vi "esp301 set home.vi"(7 "Seperator in":string, 8 "error in (no error)":errorcluster, 9 "Args":string[](array[string]), 10 "String":string, 11 "ESP301 in":refnum<class "ESP301.lvclass">) -> (0 "error out":errorcluster, 2 "new commands":string, 3 "ESP301 out":refnum<class "ESP301.lvclass">)   [LabVIEW 2020, in "ESP301.lvclass"]
uses:
  ESP301.lvclass
  ESP301.lvclass/ESP301.ctl
  shared/CompressAndUpdate(Poly)/CompressAndUpdate(Numeric).vi
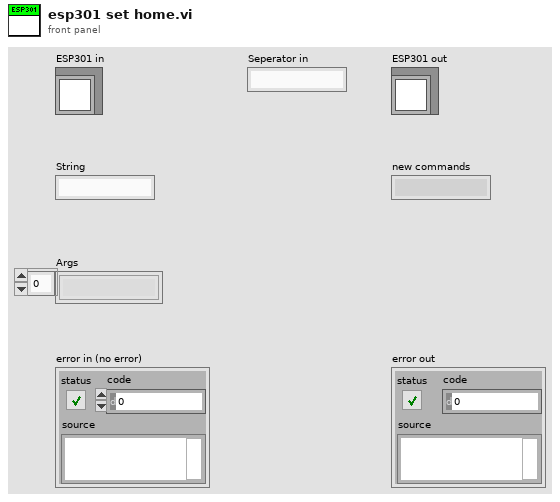
[diagram p1: front panel]
types:
  T1 = cluster{"Axis 1":cluster{"Value":dbl, "Min":dbl, "Max":dbl, "StepSize":dbl, "Tolerance":dbl, "ValueActual":dbl}, "Axis 2":cluster{"Value":dbl, "Min":dbl, "Max":dbl, "StepSize":dbl, "Tolerance":dbl, "ValueActual":dbl}, "Axis 3":cluster{"Value":dbl, "Min":dbl, "Max":dbl, "StepSize":dbl, "Tolerance":dbl, "ValueActual":dbl}}
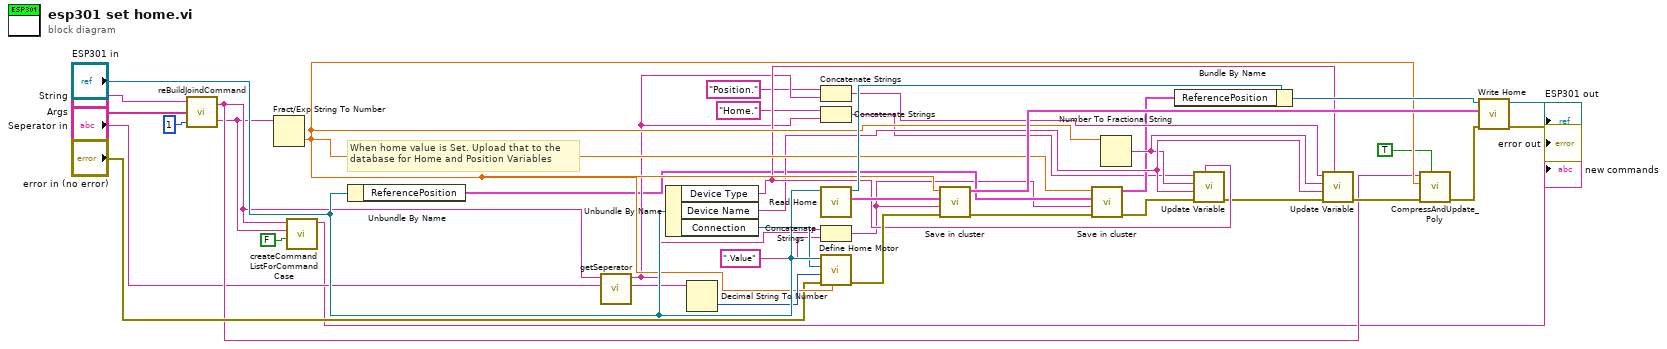
[diagram p0: block diagram]
diagram:
  # "When home value is Set. Upload that to the\ndatabase for Home and Position Variables"
  n1 = call "reBuildJoindCommand.vi"("number of group elements (0)"=1, "Args"="Args", "Command 2"="String") -> ("Arg"=w10:string, "Command"=w18:string)
  n2 = Fract/Exp String To Number(string=w10) -> (number=w28:dbl)  [unwired: 3 in, 1 out]
  n3 = call "createCommandListForCommandCase.vi"("immediate Check (only once)"=FALSE, "setvalue"=w10, "command"=w18) -> ("new commands"=→"new commands":string)  [unwired: 8 in]
  n4 = Unbundle By Name("ESP301 in") -> ("ReferencePosition"=w16:T1)
  n5 = call "getSeperator.vi"("Channel Seperator (\"\")"="Seperator in", "Command"=w18) -> ("Channel"=w8:string, "Seperator (e.g. \"Channel1\")"=w23:string)  [unwired: 8 in]
  n6 = Unbundle By Name("ESP301 in") -> ("Device Type"=w26:string, "Device Name"=w25:string, "Connection"=w29:refnum<visa-resource-name>)
  n7 = Decimal String To Number(string=w8) -> (number=w30:i32)  [unwired: 2 in, 1 out]
  n8 = Concatenate Strings("Position." ("string"), w23) -> (w22:string)
  n9 = Concatenate Strings("Home." ("string"), w23) -> (w12:string)
  n10 = call "Read Home.vi"("ESP301 in"="ESP301 in") -> ("Home"=w34:T1, "ESP301 out"=w32:refnum<class "ESP301.lvclass">)  [unwired: 8 in, 1 out]
  n11 = Concatenate Strings(w23, ".Value" ("string")) -> (w13:string)
  n12 = call-dynamic "Define Home Motor.vi"("Home Position (0 units)"=w28, "error in (no error)"="error in (no error)", "Axis (1)"=w30, "VISA resource name"=w29, "ESP301 in"="ESP301 in") -> ("error out"=w31:errorcluster)  [unwired: 4 in, 2 out]
  n13 = call "Save in cluster.vi"("error in (no error)"=w31, "String"=w13, "Home in"=w34, "Numeric"=w28) -> ("error out"=w14:errorcluster, "Home out"=w35:T1)  [unwired: 6 in]
  n14 = call "Save in cluster.vi"("error in (no error)"=w14, "String"=w13, "Home in"=w16, "Numeric"=w28) -> ("error out"=w15:errorcluster, "Home out"=w17:T1)  [unwired: 6 in]
  n15 = Number To Fractional String(number=w28) -> (F-format string=w24:string)  [unwired: 3 in]
  n16 = Bundle By Name(cluster=w32, "ReferencePosition"=w17) -> (w36:refnum<class "ESP301.lvclass">)
  n17 = call "Update Variable.vi"("Device Type"=w26, "error in (no error)"=w15, "device name"=w25, "Variable Value"=w24, "Variable Name"=w12) -> ("error out"=w19:errorcluster)  [unwired: 6 in]
  n18 = call "Update Variable.vi"("Device Type"=w26, "error in (no error)"=w19, "device name"=w25, "Variable Value"=w24, "Variable Name"=w22) -> ("error out"=w20:errorcluster)  [unwired: 6 in]
  n19 = call-poly "CompressAndUpdate_Poly.vi"("force CVT update (false)"=TRUE ("force CVT update"), "error in"=w20, "Numeric"=w28, "command or variable name"=w18) -> ("error out"=w38:errorcluster)  [unwired: 7 in]
  n20 = call "Write Home.vi"("error in (no error)"=w38, "Home"=w35, "ESP301 in"=w36) -> ("error out"=→"error out":errorcluster, "ESP301 out"=→"ESP301 out":refnum<class "ESP301.lvclass">)  [unwired: 7 in]
